vi "CPOS To Byte.vi"(11 "CPOS":T1) -> (3 "Numeric":u8)   [LabVIEW 2022 SP3, in "FHPP.lvclass"]
uses:
  FHPP.lvclass
  FHPP.lvclass/FHPP.ctl
  TypeDefs/CPOS.ctl
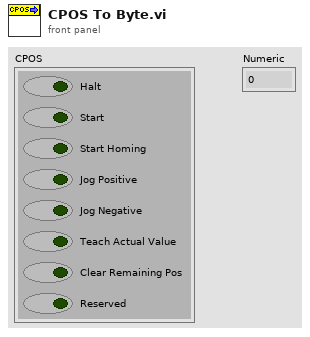
[diagram p1: front panel]
types:
  T1 = typedef "FHPP.lvclass/CPOS.ctl" = cluster{"Halt":bool, "Start":bool, "Start Homing":bool, "Jog Positive":bool, "Jog Negative":bool, "Teach Actual Value":bool, "Clear Remaining Pos":bool, "Reserved":bool}
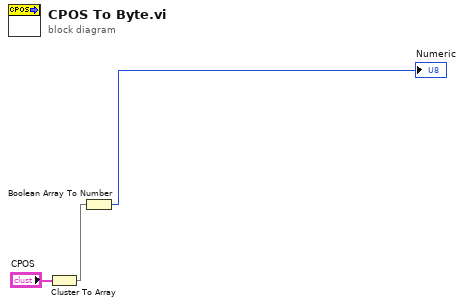
[diagram p0: block diagram]
diagram:
  n1 = Cluster To Array(cluster="CPOS") -> (array=w2:bool[])
  n2 = Boolean Array To Number(Boolean array=w2) -> (number=→"Numeric":u8)
